vi "Enable GUI Objects.vi"(8 "Error In":errorcluster, 11 "GUI Object Refs":refnum<vi>[](array[refnum])) -> (0 "Error Out":errorcluster)   [LabVIEW 2022 SP3]
doc: "<add documentation here>"
panel:
  # "Development\nControls or indicators that are useful for development or testing, but which are not outputs of the VI."
  # "Input\nInputs to the VI"
  # "Output\nOutputs of the VI"
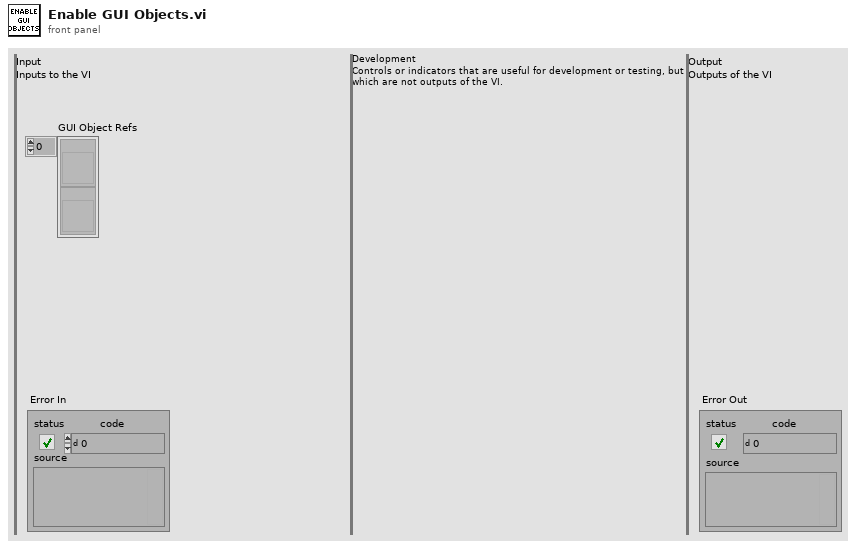
[diagram p1: front panel]
types:
  T1 = enum8{"Enabled", "Disabled", "Disabled and Grayed Out"}
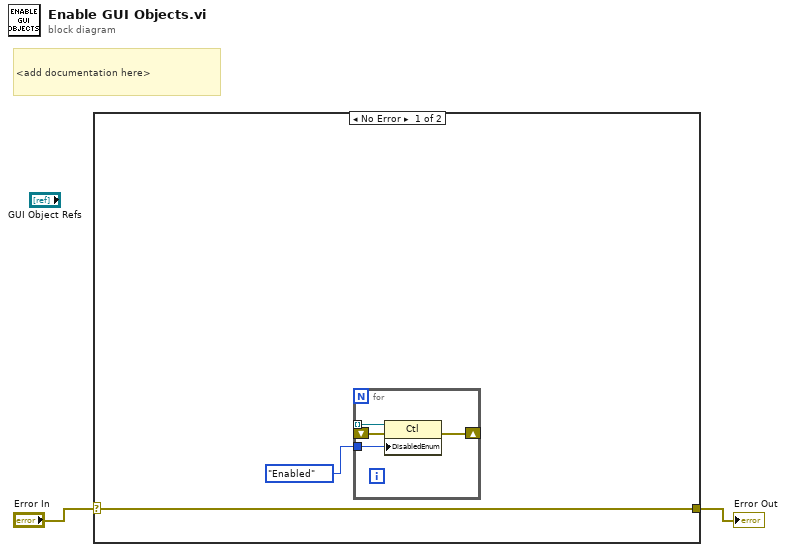
[diagram p0: block diagram]
diagram:
  # "<add documentation here>"
  n1 = case shown="No Error" "Error In" {
    selector: "Error In" -> [w6 w11]
    tunnel: [w6 w11] -> w1
    frame No Error {
      n2 = for {
        shift-right: [w9] -> _
        shift-left: [w10] -> w5
        tunnel: [w8] -> w4 mode=indexing
        tunnel: T1."Enabled" ("Disabled") -> [w7]
        n3 = property class="Ctl"(reference=w8, error in=w10, "DisabledEnum"=w7) -> (error out=w9:errorcluster)  [unwired: 1 out]
      }
    }
    frame Error {
    }
  }
  "Error Out" <- w1
